vi "Create Node String.vi"(8 "error in (no error)":errorcluster, 10 "token string":string, 11 "Is namespace or group?":bool) -> (0 "error out":errorcluster, 3 "format string":string)   [LabVIEW 2018, in "DGML creation.lvlib"]
uses:
  DGML creation.lvlib
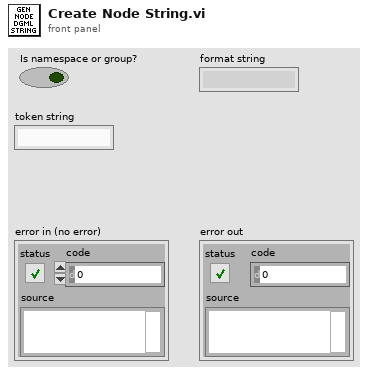
[diagram p1: front panel]
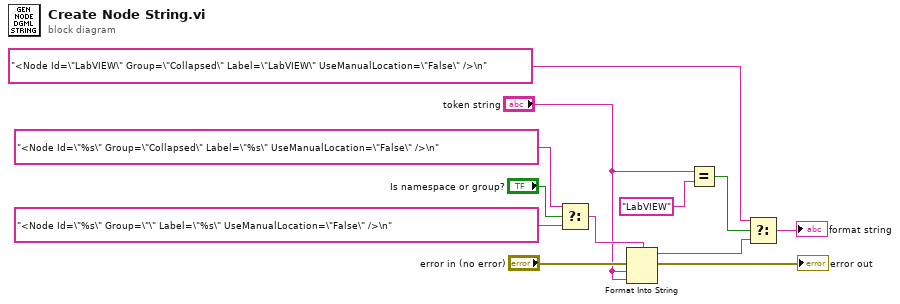
[diagram p0: block diagram]
diagram:
  n1 = Select(t="<Node Id=\"%s\" Group=\"Collapsed\" Label=\"%s\" UseManualLocation=\"False\" />\n" ("format string"), s="Is namespace or group?", f="<Node Id=\"%s\" Group=\"\" Label=\"%s\" UseManualLocation=\"False\" />\n" ("format string")) -> (s? t:f=w5:string)
  n2 = Format Into String(format string=w5, error in="error in (no error)", "token string", "token string") -> (resulting string=w6:string, error out=→"error out":errorcluster)  [unwired: 1 in]
  n3 = Equal?(x="token string", y="LabVIEW" ("regular expression")) -> (x = y?=w2:bool)
  n4 = Select(t="<Node Id=\"LabVIEW\" Group=\"Collapsed\" Label=\"LabVIEW\" UseManualLocation=\"False\" />\n" ("format string"), s=w2, f=w6) -> (s? t:f=→"format string":string)
